vi "Processing IMAQ Images Perf Test.vi"() -> ()   [LabVIEW 2022 SP3]
uses:
  778395ee-fa44-426b-b616-eba7fa786b87.vi
  53728a88-a8f8-4d8e-9b84-36c17e9fabb4.vi
  3cf7f824-373e-40f4-8729-1c08d52621fd.vi
  c80f5190-0e0a-447a-8bae-48ab6b182e28.vi
  <vilib>/Analysis/baseanly.llb/Mean (DBL).vi
  G-Embedded-Python-Interpreter-Toolkit/Null Py Object Refnum.vi
  53728a88-a8f8-4d8e-9b84-36c17e9fabb4.vi/96ddca92-7bbf-40e2-a1a5-d32f291eb6af.vi
  G-Embedded-Python-Interpreter-Toolkit-IMAQ/IMAQ to Py Object.vi/22f05568-5bba-4402-9e98-aca160827363.vi
  3cf7f824-373e-40f4-8729-1c08d52621fd.vi/6c7a13f1-33d3-431d-8188-904cac5422b3.vi
  c80f5190-0e0a-447a-8bae-48ab6b182e28.vi/6c7a13f1-33d3-431d-8188-904cac5422b3.vi
  G-Embedded-Python-Interpreter-Toolkit/Python Object Reference to Pointer Sized Ref.vi
  G-Embedded-Python-Interpreter-Toolkit/Pointer Sized Ref to Python Object Reference.vi
  G-Embedded-Python-Interpreter-Toolkit/Merge Call Library Errors.vi
  G-Embedded-Python-Interpreter-Toolkit/Generate Argument Type Info.vi
  G-Embedded-Python-Interpreter-Toolkit/Create Py Object IMAQ Image.vi
  G-Embedded-Python-Interpreter-Toolkit/G-Embedded-Python-Interpreter-Toolkit.lvlib
  G-Embedded-Python-Interpreter-Toolkit-IMAQ/G-Embedded-Python-Interpreter-Toolkit-IMAQ.lvlib
  <vilib>/Analysis/NI_AALBase.lvlib
panel:
  in  "Python Node Skip IMAQ to Array":bool
  out "GEPIT":T1(graph)
  out "GEPIT Mean":dbl format="%.5ps"
  out "Python Node Mean":dbl format="%.5ps"
  out "Python Node":T1(graph)
  out "Current Python Node Iteration":i32
  out "Current GEPIT Iteration":i32
  in  "Iterations":i32=5000
  in  "GEPIT First?":bool
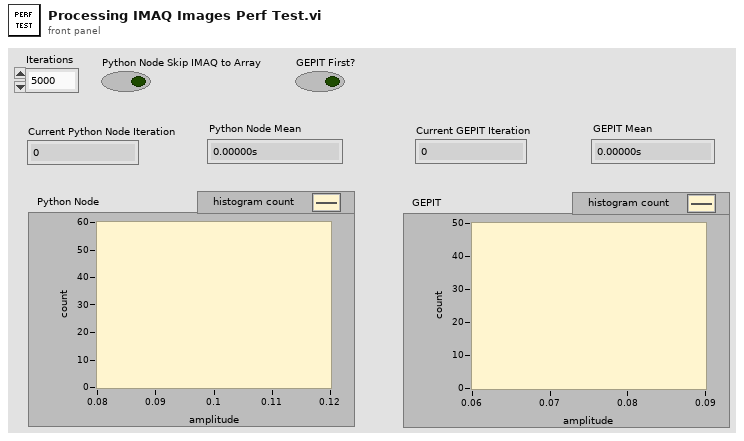
[diagram p1: front panel]
types:
  T1 = cluster{"X Values":dbl[], "Histogram: h(x)":i32[]}
  T2 = typedef "Image Type" = u32
  T3 = typedef "IMAQ Image.ctl" = refnum<image>
  T4 = typedef "G-Embedded-Python-Interpreter-Toolkit.lvlib/Python Object Reference.ctl" = refnum<k1>
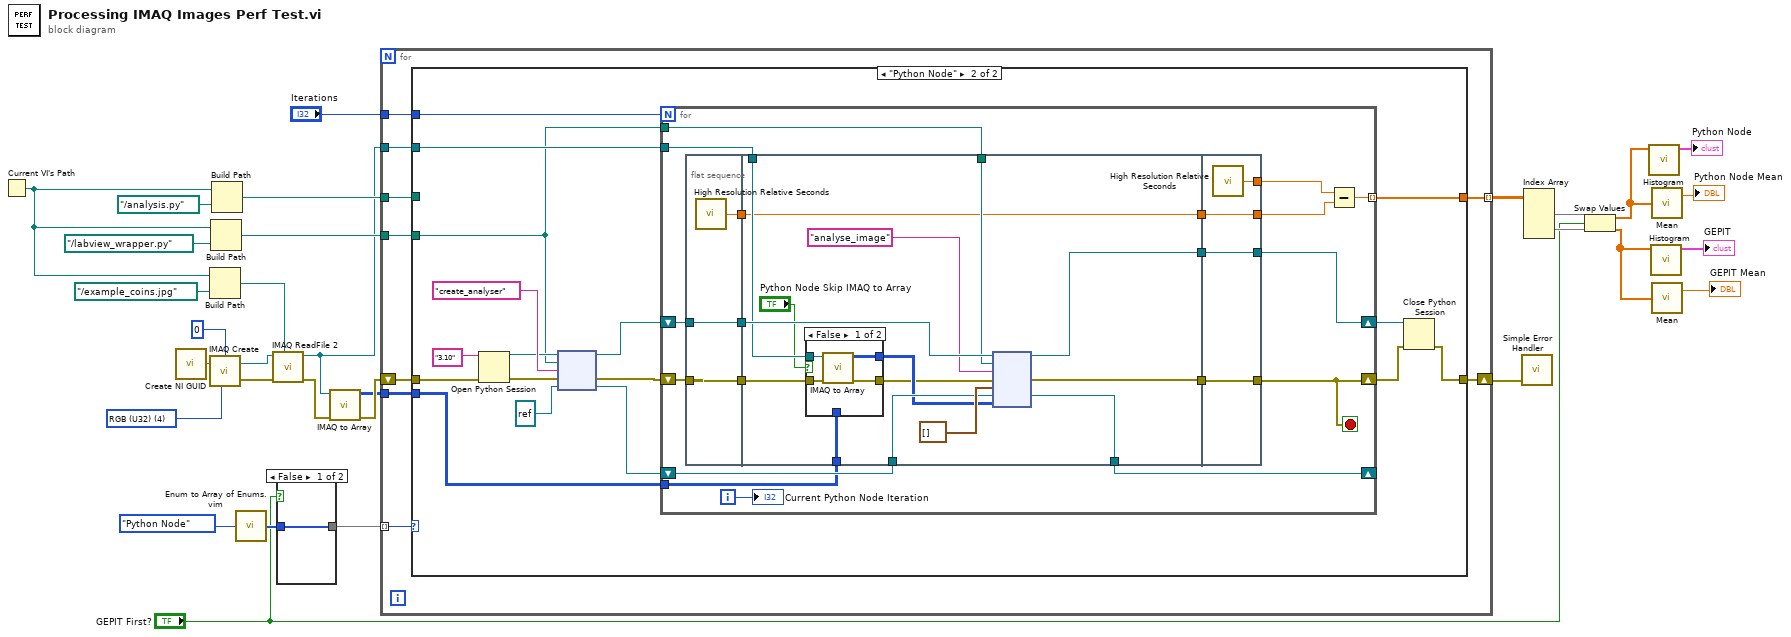
[diagram p0: block diagram]
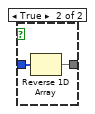
[diagram p2: hidden frame]
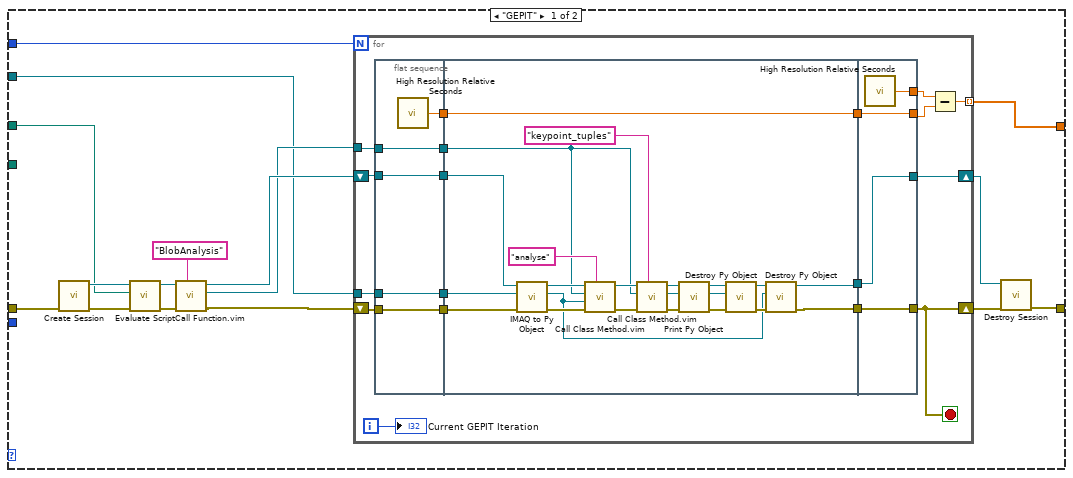
[diagram p3: hidden frame]
diagram:
  w14 = T2 4 items=["Grayscale (U8)", "Grayscale (I16)", "Grayscale (SGL)", "Complex (CSG)", "RGB (U32)", "HSL (U32)", "RGB (U64)", "Grayscale (U16)"] ("Image Type")
  n1 = Current VI's Path() -> (path=w19:path)
  n2 = call <vilib>:"Create NI GUID.vi"() -> ("NI GUID"=w17:string)
  n3 = Build Path(base path=w19, name or relative path=path "../example_coins.jpg") -> (appended path=w12:path)
  n4 = call "IMAQ Create"("Border Size"=0, "Image Name"=w17, "Image Type"=w14) -> ("New Image"=w16:T3, "error out"=w13:errorcluster)  [unwired: 2 in]
  n5 = Build Path(base path=w19, name or relative path=path "../labview_wrapper.py" ("module path")) -> (appended path=w11:path)
  n6 = Build Path(base path=w19, name or relative path=path "../analysis.py") -> (appended path=w20:path)
  n7 = call "Enum to Array of Enums.vim"("enum"=enum16{"Python Node", "GEPIT"}."Python Node") -> ("array of enums"=w30:enum16{"Python Node", "GEPIT"}[])
  n8 = call "IMAQ ReadFile 2"("File Path"=w12, "error in (no error)"=w13, "Image"=w16) -> ("error out"=w4:errorcluster, "Image Out"=w3:T3)  [unwired: 4 in, 3 out]
  n9 = case shown="False" "GEPIT First?" {
    tunnel: w30 -> [w32 w34]
    tunnel: [w32 w33] -> w29
    frame False {
    }
    frame True {
      n10 = Reverse 1D Array(array=w34) -> (reversed array=w33:enum16{"Python Node", "GEPIT"}[])
    }
  }
  n11 = call "IMAQ to Array.vi"("error in (no error)"=w4, "Refnum in"=w3) -> ("error out"=w2:errorcluster, "Array"=w1:u8[][][])  [unwired: 8 in]
  n12 = for {
    tunnel: w29 -> [w43] mode=indexing
    shift-right: [w42] -> w28
    shift-left: w2 -> [w41]
    tunnel: "Iterations" -> [w40]
    tunnel: [w39] -> w26 mode=indexing
    tunnel: w20 -> [w38]
    tunnel: w3 -> [w37]
    tunnel: w11 -> [w36]
    tunnel: w1 -> [w35]
    n13 = case shown="\"Python Node\"" w43 {
      tunnel: [w46 w113] -> w42
      tunnel: w41 -> [w52 w119]
      tunnel: w40 -> [w51 w125]
      tunnel: [w50 w124] -> w39
      tunnel: w38 -> [w49 _]
      tunnel: w37 -> [w45 w112]
      tunnel: w36 -> [_ w111]
      tunnel: w35 -> [_ w109]
      frame "GEPIT" {
        n14 = call "Create Session.vi"("error in (no error)"=w52) -> ("error out"=w59:errorcluster, "Session Handle"=w58:refnum<data-value>)  [unwired: 9 in]
        n15 = call "Evaluate Script.vi"("error in (no error)"=w59, "Script File Path"=w49, "Session Handle in"=w58) -> ("error out"=w55:errorcluster, "Session Handle out"=w56:refnum<data-value>)  [unwired: 7 in]
        n16 = call "Call Function.vim"("Function Name"="BlobAnalysis", "error in (no error)"=w55, "Data Value Reference in"=w56) -> ("error out"=w44:errorcluster, "Returned Python Object Refnum"=w53:T4, "Data Value Reference out"=w54:refnum<data-value>)  [unwired: 6 in]
        n17 = for {
          N: w51 -> [_]
          tunnel: w53 -> [w74]
          tunnel: w45 -> [w75]
          shift-right: [w63] -> w48
          shift-left: w44 -> [w76]
          tunnel: [w68] -> w50 mode=indexing
          shift-right: [w65] -> w47
          shift-left: w54 -> [w77]
          i -> [w67]
          stop <- w63 stop-if-true
          n18 = flat-sequence {
            tunnel: w74 -> [w79]
            tunnel: w75 -> [w80]
            tunnel: w76 -> [w81]
            tunnel: w77 -> [w82]
            tunnel: [w82] -> w73
            tunnel: [w81] -> w72
            tunnel: [w80] -> w71
            tunnel: [w79] -> w70
            tunnel: [w78] -> w61
            tunnel: w73 -> [w103]
            tunnel: w72 -> [w102]
            tunnel: w71 -> [w92]
            tunnel: w70 -> [w86]
            tunnel: [w85] -> w66
            tunnel: [w84] -> w64
            tunnel: [w83] -> w62
            tunnel: w61 -> [w83]
            tunnel: [w108] -> w69
            tunnel: [w107] -> w65
            tunnel: w66 -> [w107]
            tunnel: [w106] -> w63
            tunnel: w64 -> [w106]
            tunnel: [w105] -> w60
            tunnel: w62 -> [w105]
            frame #0 {
              n19 = call <vilib>:"High Resolution Relative Seconds.vi"() -> ("relative seconds"=w78:dbl)
            }
            frame #1 {
              n20 = call "IMAQ to Py Object.vi"("error in (no error)"=w102, "Image In"=w92, "Session Handle in"=w103) -> ("error out"=w100:errorcluster, "Python Object Refnum"=w87:T4, "Session Handle out"=w101:refnum<data-value>)  [unwired: 6 in]
              n21 = call "Call Class Method.vim"("Function Name"="analyse", "error in (no error)"=w100, "Arguments in (Default - Empty)"=w87, "Class Instance"=w86, "Data Value Reference in"=w101) -> ("error out"=w99:errorcluster, "Data Value Reference out"=w95:refnum<data-value>)  [unwired: 4 in, 1 out]
              n22 = call "Call Class Method.vim"("Function Name"="keypoint_tuples", "error in (no error)"=w99, "Class Instance"=w86, "Data Value Reference in"=w95) -> ("error out"=w98:errorcluster, "Returned Python Object Refnum"=w96:T4, "Data Value Reference out"=w94:refnum<data-value>)  [unwired: 5 in]
              n23 = call "Print Py Object.vi"("error in (no error)"=w98, "Python Object Refnum in"=w96, "Session Handle in"=w94) -> ("error out"=w93:errorcluster, "Python Object Refnum out"=w90:T4, "Session Handle out"=w91:refnum<data-value>)  [unwired: 5 in, 1 out]
              n24 = call "Destroy Py Object.vi"("error in (no error)"=w93, "Python Object Refnum"=w90, "Session Handle in"=w91) -> ("error out"=w89:errorcluster, "Session Handle out"=w88:refnum<data-value>)  [unwired: 7 in]
              n25 = call "Destroy Py Object.vi"("error in (no error)"=w89, "Python Object Refnum"=w87, "Session Handle in"=w88) -> ("error out"=w84:errorcluster, "Session Handle out"=w85:refnum<data-value>)  [unwired: 7 in]
            }
            frame #2 {
              n26 = call <vilib>:"High Resolution Relative Seconds.vi"() -> ("relative seconds"=w108:dbl)
            }
          }
          n27 = Subtract(x=w69, y=w60) -> (x-y=w68:dbl)
          "Current GEPIT Iteration" <- w67
        }
        n28 = call "Destroy Session.vi"("error in (no error)"=w48, "Session Handle"=w47) -> ("error out"=w46:errorcluster)  [unwired: 9 in]
      }
      frame "Python Node" {
        n29 = Open Python Session(python version="3.10" ("Python version"), 3:w119) -> (session out=w118:refnum<k35>, error out=w123:errorcluster)  [unwired: 1 in]
        n30 = node(w118, w111, "create_analyser" ("function name"), w123, refnum<k38> refnum ("Python Object Refnum")) -> (w117:refnum<k35>, w110:errorcluster, w116:refnum<k38>)  [unwired: 2 out]
        n31 = for {
          N: w125 -> [_]
          shift-right: [w132] -> w114
          shift-left: w110 -> [w144]
          tunnel: [w141] -> w124 mode=indexing
          shift-right: [w137] -> w115
          shift-left: w117 -> [w138]
          tunnel: w111 -> [w134]
          tunnel: w112 -> [w131]
          shift-right: [w127] -> _
          shift-left: w116 -> [w135]
          tunnel: w109 -> [w126]
          i -> [w140]
          stop <- w132 stop-if-true
          n32 = flat-sequence {
            tunnel: w144 -> [w147]
            tunnel: [w147] -> w143
            tunnel: [w146] -> w139
            tunnel: w138 -> [w146]
            tunnel: [w145] -> w129
            tunnel: w143 -> [w160]
            tunnel: w139 -> [w162]
            tunnel: [w161] -> w136
            tunnel: w135 -> [w158]
            tunnel: w134 -> [w155]
            tunnel: [w153] -> w133
            tunnel: w131 -> [w152]
            tunnel: [w151] -> w130
            tunnel: w129 -> [w151]
            tunnel: [w150] -> w127
            tunnel: w126 -> [w149]
            tunnel: [w172] -> w142
            tunnel: [w171] -> w137
            tunnel: w136 -> [w171]
            tunnel: [w170] -> w132
            tunnel: w133 -> [w170]
            tunnel: w130 -> [w169]
            tunnel: [w169] -> w128
            frame #0 {
              n33 = call <vilib>:"High Resolution Relative Seconds.vi"() -> ("relative seconds"=w145:dbl)
            }
            frame #1 {
              n34 = case shown="False" "Python Node Skip IMAQ to Array" {
                tunnel: w160 -> [w166 w167]
                tunnel: [w165 w168] -> w157
                tunnel: [w164 w167] -> w156
                tunnel: w152 -> [w163 _]
                tunnel: w149 -> [_ w168]
                frame False {
                  n35 = call "IMAQ to Array.vi"("error in (no error)"=w166, "Refnum in"=w163) -> ("error out"=w164:errorcluster, "Array"=w165:u8[][][])  [unwired: 8 in]
                }
                frame True {
                }
              }
              n36 = node(w162, w155, "analyse_image" ("function name"), w156, cluster{"x":i32, "y":i32, "diameter":i32}[] [], w158, w157) -> (w161:refnum<k35>, w153:errorcluster, w150:refnum<k38>)  [unwired: 2 in, 2 out]
            }
            frame #2 {
              n37 = call <vilib>:"High Resolution Relative Seconds.vi"() -> ("relative seconds"=w172:dbl)
            }
          }
          n38 = Subtract(x=w142, y=w128) -> (x-y=w141:dbl)
          "Current Python Node Iteration" <- w140
        }
        n39 = Close Python Session(session in=w115, error in=w114) -> (11:w113:errorcluster)
      }
    }
  }
  n40 = call <vilib>:"Simple Error Handler.vi"("error in (no error)"=w28) -> ()  [unwired: 4 in, 5 out]
  n41 = Index Array(array=w26) -> (element #1=w25:dbl[], element #2=w24:dbl[])  [unwired: 4 in]
  n42 = Swap Values(12:w25, 13:"GEPIT First?", 14:w24) -> (1:w9:dbl[], 3:w7:dbl[])
  n43 = call <vilib>:"Histogram.vi"("X"=w9) -> ("Histogram Graph"=→"Python Node":T1)  [unwired: 7 in, 3 out]
  n44 = call <vilib>:"Histogram.vi"("X"=w7) -> ("Histogram Graph"=→"GEPIT":T1)  [unwired: 7 in, 3 out]
  n45 = call-poly <vilib>:"Mean.vi"("X"=w9) -> ("mean"=→"Python Node Mean":dbl)  [unwired: 1 out]
  n46 = call-poly <vilib>:"Mean.vi"("X"=w7) -> ("mean"=→"GEPIT Mean":dbl)  [unwired: 1 out]
